vi "EnableDualPass.vi"(8 "error in":T2, 11 "Dual Pass State":T1=-2147483648 items=["[read only]"=-2147483648, "No"=0, "Yes"=1]) -> (0 "error out":T2, 3 "Dual Pass State out":T1=-2147483648 items=["[read only]"=-2147483648, "No"=0, "Yes"=1])   [LabVIEW 2016]
doc: "Activates (state = 1) or deactivates (state = 0) the dual pass mode."
uses:
  Controls/Error_Out.ctl
  Controls/Dual-Pass-State_Selection.ctl
  Files_ASC500/DLL/ASC500_RemoteControlV27.dll
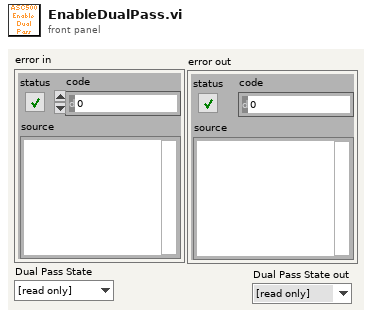
[diagram p1: front panel]
types:
  T1 = typedef "Dual-Pass-State_Selection.ctl" = i32
  T2 = typedef "Error_Out.ctl" = errorcluster
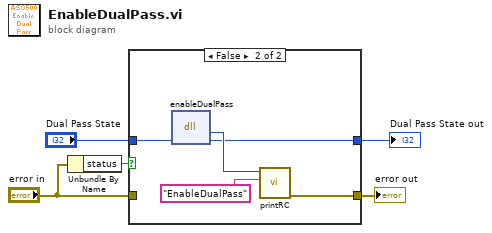
[diagram p0: block diagram]
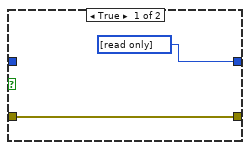
[diagram p2: hidden frame]
diagram:
  n1 = Unbundle By Name("error in") -> ("status"=w5:bool)
  n2 = case shown="False" w5 {
    tunnel: [w7 w11] -> w4
    tunnel: "Dual Pass State" -> [_ w12]
    tunnel: "error in" -> [w7 _]
    tunnel: [w6 w8] -> w1
    frame True {
      w6 = T1 -2147483648 items=["[read only]"=-2147483648, "No"=0, "Yes"=1] ("Dual Pass State out")
    }
    frame False {
      n3 = dll-call lib="G:/SCMOperations/Share/ELE/Produkt Information/ASC500/04 Remote Control/02 development versions/2018Nov06/Files_ASC500/DLL/ASC500_RemoteControlV27.dll" fn="enableDualPass"("State"=w12) -> ("return type"=w10:i32, "State"=w8:i32)  [unwired: 3 in, 2 out]
      n4 = call "printRC.vi"("additional information"="EnableDualPass", "RC"=w10) -> ("error out"=w11:T2)  [unwired: 9 in]
    }
  }
  "error out" <- w4
  "Dual Pass State out" <- w1
